vi "Get Team Index.vi"(8 "error in (no error)":errorcluster, 11 "Team Dashboard Panel in":refnum<class "Team Dashboard Panel.lvclass">) -> (0 "error out":errorcluster, 2 "Team Index":i32, 3 "Team Dashboard Panel out":refnum<class "Team Dashboard Panel.lvclass">)   [LabVIEW 2020, in "SB App.lvlib" / "Team Dashboard Panel.lvclass"]
uses:
  Team Dashboard Panel.lvclass
  Team Dashboard Panel.lvclass/Team Dashboard Panel.ctl
  SquareBattle/Team/Team.lvclass
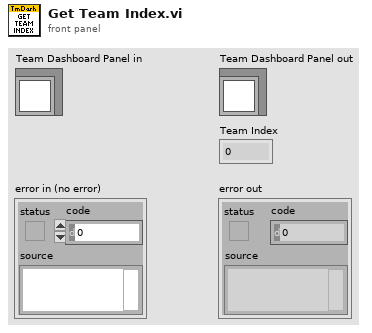
[diagram p1: front panel]
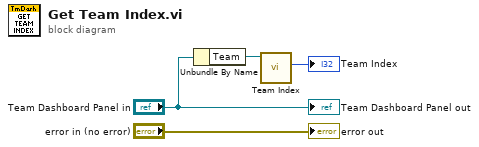
[diagram p0: block diagram]
diagram:
  n1 = Unbundle By Name("Team Dashboard Panel in") -> ("Team"=w2:refnum<class "Team.lvclass">)
  n2 = call "Team Index.vi"("Team"=w2) -> ("Team Index"=→"Team Index":i32)  [unwired: 10 in]
  "error out" <- "error in (no error)"
  "Team Dashboard Panel out" <- "Team Dashboard Panel in"
